vi "BMark_Rect Width and Height.vi"(11 "Rectangle":T1) -> (0 "Vert Center":i16, 1 "Horiz Center":i16, 2 "Height":i16, 3 "Width":i16)   [LabVIEW 2013]
uses:
  <vilib>/Utility/miscctls.llb/LVRectTypeDef.ctl
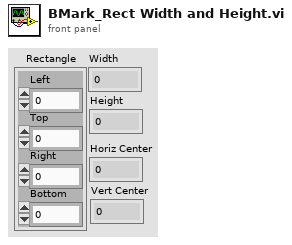
[diagram p1: front panel]
types:
  T1 = typedef "LVRectTypeDef.ctl" = cluster{"Left":i16, "Top":i16, "Right":i16, "Bottom":i16}
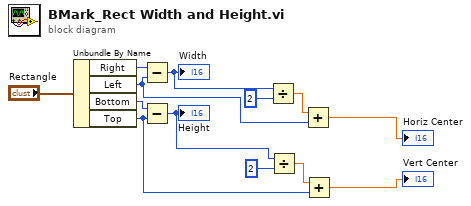
[diagram p0: block diagram]
diagram:
  n1 = Unbundle By Name("Rectangle") -> ("Right"=w12:i16, "Left"=w7:i16, "Bottom"=w11:i16, "Top"=w3:i16)
  n2 = Subtract(x=w12, y=w7) -> (x-y=w10:i16)
  "Width" <- w10
  n3 = Subtract(x=w11, y=w3) -> (x-y=w4:i16)
  "Height" <- w4
  n4 = Divide(x=w10, y=i16 2) -> (x/y=w8:dbl)
  n5 = Divide(x=w4, y=i16 2) -> (x/y=w6:dbl)
  n6 = Add(x=w8, y=w7) -> (x+y=→"Horiz Center":dbl)
  n7 = Add(x=w6, y=w3) -> (x+y=→"Vert Center":dbl)
